vi "Define Columns.vi"(10 "Enum Array":refnum<vi>[](array[refnum])) -> (2 "Column Definition":T1[](array[typedef]) {"MinWidth" min=2 step=1; "AutoSizeMode" items=["None"=1, "ColumnHeader"=2, "AllCellsExceptHeader"=4, "AllCells"=6, "DisplayedCellsExceptHeader"=8, "DisplayedCells"=10, "Fill"=16]; "FillWeight" min=1 max=100})   [LabVIEW 2013, in "tag bus configurable plugin editor node.lvclass"]
uses:
  tag bus configurable plugin editor node.lvclass
  <vilib>/NI/DCAF Table API/Column/Column Descriptor.ctl
  <vilib>/NI/DCAF Table API/Column/Column Type.ctl
  <vilib>/NI/Tag Bus/tag/Data Type.ctl
  <vilib>/NI/DCAF Table API/Table Manager/Call Back Ref Type Def.ctl
  <vilib>/NI/DCAF/Tag Editor Core/Configuration Editor/Classes/Engine Parent/Engine Parent Editor Node.lvclass
  <vilib>/NI/DCAF/Tag Editor Core/Configuration Editor/Classes/Module editor node/module editor node.lvclass
  Callback Change Channel Name.vi
  Callback Change Data Type.vi
  Callback Change Tag.vi
  Callback Change Direction.vi
  <vilib>/NI/DCAF Table API/Column/Column.lvclass
  <vilib>/NI/Tag Bus/tag/tag descriptor.lvclass
  <vilib>/NI/DCAF Table API/Table Manager/Table Manager.lvclass
  <vilib>/NI/DCAF Table API/Mapping Column/Mapping Column.lvclass
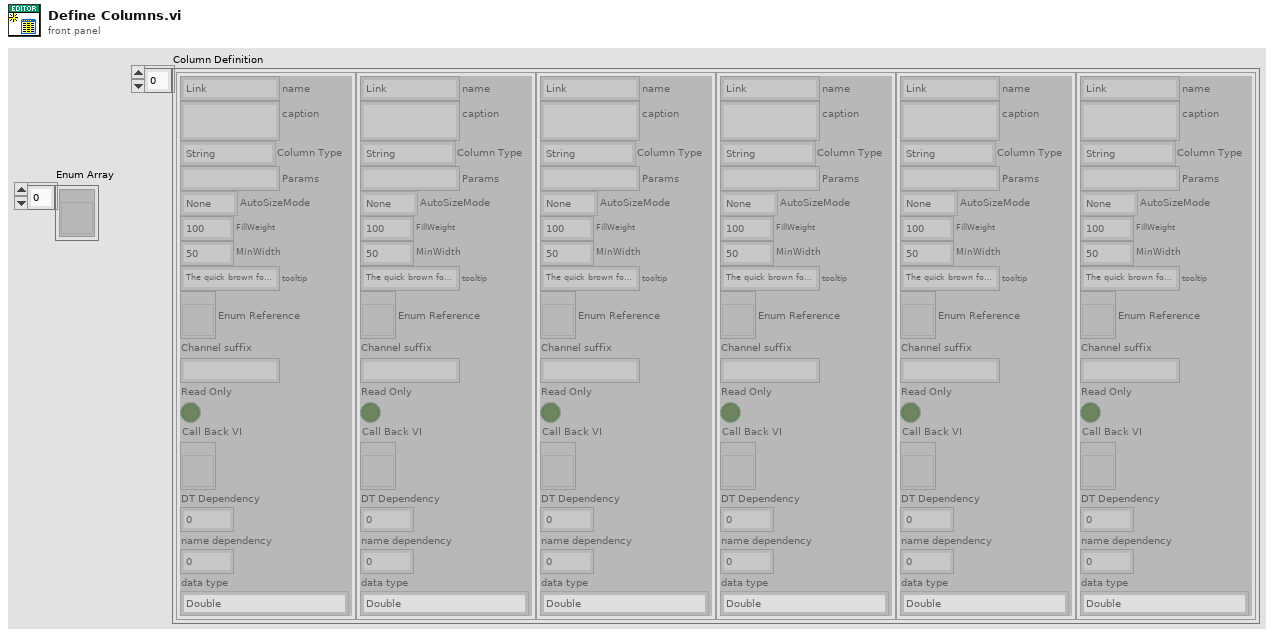
[diagram p1: front panel]
types:
  T1 = typedef "Table Manager.lvlib/Column.lvclass/Column Descriptor.ctl" = cluster{"name":string, "caption":string, "Column Type":T2, "Params":string, "AutoSizeMode":i32, "FillWeight":sgl, "MinWidth":u32, "tooltip":string, "Enum Reference":refnum<vi>, "Channel suffix":string, "Read Only":bool, "Call Back VI":T3, "DT Dependency":i32, "name dependency":i32, "data type":T4}
  T2 = typedef "Table Manager.lvlib/Column.lvclass/Column Type.ctl" = enum16{"String", "Mapping", "Channel Name", "Tag", "Enum", "Data Type", "Numeric"}
  T3 = typedef "Table Manager.lvlib/Table Manager.lvclass/Call Back Ref Type Def.ctl" = refnum<vi>
  T4 = typedef "tag bus.lvlib/tag descriptor.lvclass/Data Type.ctl" = enum16{"Double", "Single", "I64", "I32", "I16", "I8", "U64", "U32", "U16", "U8", "Boolean", "String", "Array of Double", "Array of Single", "Array of I64", "Array of I32", "Array of I16", "Array of I8", "Array of U64", "Array of U32", "Array of U16", "Array of U8", "Array of Boolean", "Array of String"}
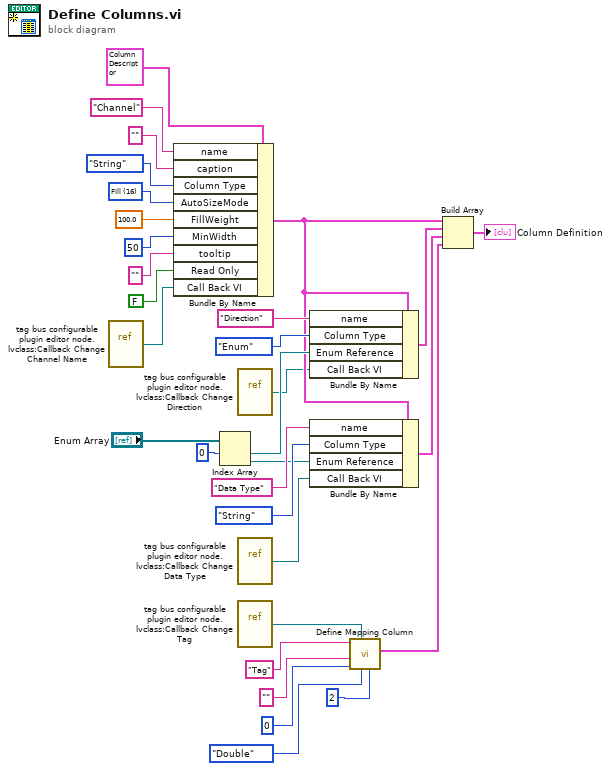
[diagram p0: block diagram]
diagram:
  w20 = 16 items=["None"=1, "ColumnHeader"=2, "AllCellsExceptHeader"=4, "AllCells"=6, "DisplayedCellsExceptHeader"=8, "DisplayedCells"=10, "Fill"=16] ("AutoSizeMode")
  n1 = vi-ref "tag bus configurable plugin editor node.lvclass:Callback Change Channel Name.vi"() -> (w17:refnum<vi>)
  n2 = Bundle By Name(cluster=T1 {"name"="", "caption"="", "Column Type"=enum."String", "Params"="", "AutoSizeMode"=0, "FillWeight"=0.0, "MinWidth"=0, "tooltip"="", "Enum Reference"=refnum, "Channel suffix"="", "Read Only"=FALSE, "Call Back VI"=refnum, "DT Dependency"=0, "name dependency"=0, "data type"=enum."Double"} ("Table Manager.lvlib:Column.lvclass:Column Descriptor"), "name"="Channel", "caption"="", "Column Type"=Column_Type."String", "AutoSizeMode"=w20, "FillWeight"=sgl 100.0, "MinWidth"=u32 50, "tooltip"="", "Read Only"=FALSE, "Call Back VI"=w17) -> (w10:T1)
  n3 = Index Array(array="Enum Array", index #1=0 ("index")) -> (element #1=w27:refnum<vi>, element #2=w5:refnum<vi>)  [unwired: 1 in]
  n4 = vi-ref "tag bus configurable plugin editor node.lvclass:Callback Change Direction.vi"() -> (w3:refnum<vi>)
  n5 = vi-ref "tag bus configurable plugin editor node.lvclass:Callback Change Data Type.vi"() -> (w4:refnum<vi>)
  n6 = vi-ref "tag bus configurable plugin editor node.lvclass:Callback Change Tag.vi"() -> (w16:refnum<vi>)
  n7 = Bundle By Name(cluster=w10, "name"="Direction", "Column Type"=Column_Type."Enum", "Enum Reference"=w27, "Call Back VI"=w3) -> (w31:T1)
  n8 = Bundle By Name(cluster=w10, "name"="Data Type", "Column Type"=Column_Type."String", "Enum Reference"=w5, "Call Back VI"=w4) -> (w9:T1)
  n9 = call <vilib>:"Define Mapping Column.vi"("DT Dependency"=2, "data type"=Data_Type."Double", "Call Back VI"=w16, "name dependency"=0, "Channel suffix"="" ("string"), "name"="Tag") -> ("Table Manager.lvlib:Column.lvclass:Column Descriptor"=w6:T1)  [unwired: 5 in]
  n10 = Build Array(w10, w31, w9, w6) -> (→"Column Definition":T1[])
